vi "Zadanie_3.1.vi"() -> ()   [LabVIEW 2021]
panel:
  out "Liczby losowe":dbl(graph)
  in  "stop":bool
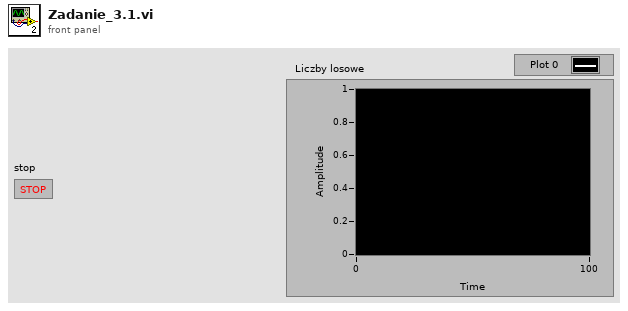
[diagram p1: front panel]
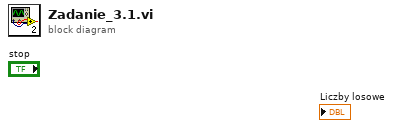
[diagram p0: block diagram]
diagram:
